vi "Unpack for gRPC.vi"(8 "error in":errorcluster, 9 "configuration / results":enum16{"Configuration", "Results"}(ring), 10 "any":T1, 11 "measurement plugin in":refnum<class "FPT Intermodulation.lvclass">) -> (0 "error out":errorcluster, 2 "data value":variant, 3 "measurement plugin out":refnum<class "FPT Intermodulation.lvclass">)   [LabVIEW 2023, in "FPT Intermodulation.lvclass"]
uses:
  FPT Intermodulation.lvclass
  <vilib>/gRPC/LabVIEW gRPC Library/Shared/Any.ctl
  C:/Program Files/National Instruments/LabVIEW 2023/vi.lib/Plug-In SDKs/Measurements/Measurement Plugin Service/Measurement Plugin Service.lvclass
  Measurement Configuration.ctl
  Measurement Results.ctl
  a521b266-ce99-437c-923d-067dcf1e07fd.vi
  3ecd018e-d556-4cbc-bc60-c4ba57204520.vi
  <vilib>/gRPC/LabVIEW gRPC Library/Server API/Translate Protobuf Error.vi
  <vilib>/AdvancedString/1D String Array to Delimited String.vi
  <vilib>/gRPC/LabVIEW gRPC Library/Server API/Server/Get Server DLL Path.vi
  <vilib>/Plug-In SDKs/Measurements/Measurement Plugin Service/Measurement Plugin Service.lvclass
  <vilib>/gRPC/LabVIEW gRPC Library/grpc-lvsupport-release.lvlib
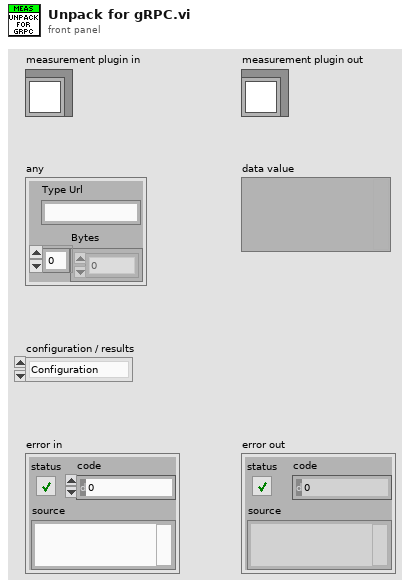
[diagram p1: front panel]
types:
  T1 = typedef "grpc-lvsupport-release.lvlib/Any.ctl" = cluster{"Type Url":string, "Bytes":u8[]}
  T2 = typedef "grpc-lvsupport-release.lvlib/grpcId.ctl" = u64
  T3 = typedef "FPT Intermodulation.lvclass/Measurement Configuration.ctl" = cluster{"Automation Test":bool, "Power sequencing file path":string, "RFSG name":string, "RFSG port":string, "RFSG attenuation mode":enum32{"<None>", "Constant Attenuation", "s2p File"}, "RFSG external attenuation (dB)":dbl, "RFSG s-parameters orientation":enum32{"Port1 Towards DUT", "Port2 Towards DUT"}, "RFSG s2p file path":string, "RFmx name":string, "RFmx port":string, "RFmx attenuation mode":enum32{"<None>", "Constant Attenuation", "s2p File"}, "RFmx external attenuation (dB)":dbl, "RFmx s-parameters orientation":enum32{"Port1 Towards DUT", "Port2 Towards DUT"}, "RFmx s2p file path":string, "RFmx Reference Level (dBm)":dbl, "RFSG Generation IQ Rate (S/s)":dbl, "Target Pout Per Tone (dBm)":dbl, "Start Pin Per Tone (dBm)":dbl, "Start Center Frequency (Hz)":dbl, "Start Tone Spacing (Hz)":dbl, "IM_Sweep Mode":enum32{"Power", "Frequency", "Tone Spacing"}, "Sweep Delay (ms)":u32, "Power Sweep End":dbl, "Power Sweep Step":dbl, "Frequency Sweep End":dbl, "Frequency Sweep Step":dbl, "Tone Spacing Sweep End":dbl, "Tone Spacing Sweep Step":dbl}
  T4 = typedef "FPT Intermodulation.lvclass/Measurement Results.ctl" = cluster{"Status":string, "Typical OIP3 (dBm)":dbl, "TS_Fundamental (dBm)":dbl[][], "TS_IMD (dBm)":dbl[][], "TS_TOI (dBm)":dbl[][], "TS_DUT Gain (dBm)":dbl[][], "Final Target Pout (dBm)":dbl}
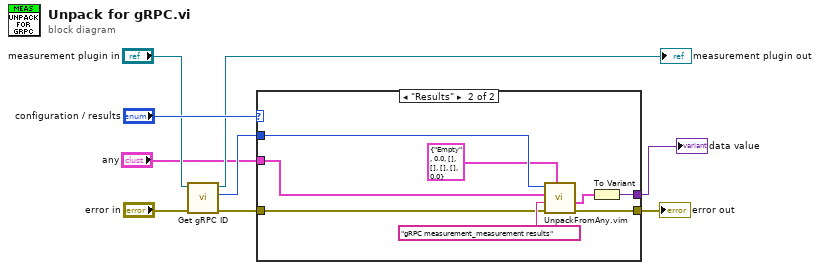
[diagram p0: block diagram]
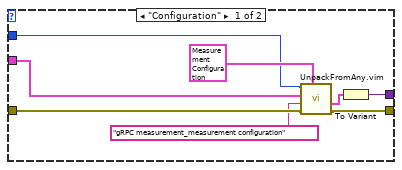
[diagram p2: hidden frame]
diagram:
  n1 = call <vilib>:"Get gRPC ID.vi"("error in"="error in", "measurement plugin service in"="measurement plugin in") -> ("error out"=w6:errorcluster, "gRPC ID"=w3:T2, "measurement plugin service out"=→"measurement plugin out":refnum<class "FPT Intermodulation.lvclass">)  [unwired: 7 in]
  n2 = case shown="\"Results\"" "configuration / results" {
    tunnel: w6 -> [w15 w19]
    tunnel: "any" -> [w10 w18]
    tunnel: w3 -> [w12 w22]
    tunnel: [w16 w23] -> w9
    tunnel: [w17 w25] -> w1
    frame "Configuration" {
      n3 = call "UnpackFromAny.vim"("Data Type"=T3 {"Automation Test"=FALSE, "Power sequencing file path"="Lorem ipsum dolor sit", "RFSG name"="5842_0", "RFSG port"="", "RFSG attenuation mode"=enum."Constant Attenuation", "RFSG external attenuation (dB)"=32.0, "RFSG s-parameters orientation"=enum."Port2 Towards DUT", "RFSG s2p file path"="", "RFmx name"="5842_0", "RFmx port"="", "RFmx attenuation mode"=enum."<None>", "RFmx external attenuation (dB)"=1.0, "RFmx s-parameters orientation"=enum."Port2 Towards DUT", "RFmx s2p file path"="", "RFmx Reference Level (dBm)"=10.0, "RFSG Generation IQ Rate (S/s)"=1250000000.0, "Target Pout Per Tone (dBm)"=10.0, "Start Pin Per Tone (dBm)"=10.0, "Start Center Frequency (Hz)"=10.0, "Start Tone Spacing (Hz)"=10.0, "IM_Sweep Mode"=enum."Power", "Sweep Delay (ms)"=10, "Power Sweep End"=10.0, "Power Sweep Step"=10.0, "Frequency Sweep End"=-4.0, "Frequency Sweep Step"=1.0, "Tone Spacing Sweep End"=-4.0, "Tone Spacing Sweep Step"=1.0} ("Measurement Configuration"), "error in"=w15, "Message Type"="gRPC measurement_measurement configuration", "Any"=w10, "gRPCid in"=w12) -> ("error out"=w16:errorcluster, "Unpacked Value"=w14:T3)  [unwired: 4 in, 1 out]
      n4 = To Variant(anything=w14) -> (Variant=w17:variant)
    }
    frame "Results" {
      n5 = call "UnpackFromAny.vim"("Data Type"=T4 {"Status"="Empty", "Typical OIP3 (dBm)"=0.0, "TS_Fundamental (dBm)"=[], "TS_IMD (dBm)"=[], "TS_TOI (dBm)"=[], "TS_DUT Gain (dBm)"=[], "Final Target Pout (dBm)"=0.0} ("Measurement Results"), "error in"=w19, "Message Type"="gRPC measurement_measurement results", "Any"=w18, "gRPCid in"=w22) -> ("error out"=w23:errorcluster, "Unpacked Value"=w24:T4)  [unwired: 4 in, 1 out]
      n6 = To Variant(anything=w24) -> (Variant=w25:variant)
    }
  }
  "error out" <- w9
  "data value" <- w1
